vi "SVFA Get Tone Amplitude and Phase (1 Ch).vi"(0 "complex spectrum":T8={"complex spectrum response"={"f0"=0.0, "df"=1.0, "complex spectrum"=[]}, "spectrum info"={"channel name"="", "description"="", "x-axis units"=0, "spectral info"={"spectrum type"=enum."Power [Magnitude^2]", "linear/dB"=enum."linear", "window"=0, "window size"=0, "FFT size"=0}, "engineering units"=0, "custom label"="", "dB reference [EU]"=0.0, "peak units"=enum."rms", "weighting filter"=0, "spectral density?"=FALSE, "unit label"="", "spectrum skewed?"=FALSE, "complimentary spectrum units"=enum."none"}} {"spectrum info"."x-axis units" items=["Time (s)"=0, "Frequency-CB (Hz)"=1, "Frequency-CPB (Hz)"=1248, "Frequency-Arbitrary (Hz)"=2357, "Quefrency (s)"=2, "Revolutions (rev)"=3, "Order"=4, "Speed (RPM)"=11, "Speed (rad/s)"=21, "Index"=65535]; "spectrum info"."weighting filter" items=["Linear", "A-weighting", "B-weighting", "C-weighting", "ITU-R 468-4", "Dolby", "CCITT", "C-message", "Wb", "Wc", "Wd", "We", "Wf", "Wh", "Wj", "Wk", "Wm", "AES17 20 kHz lowpass", "AES17 40 kHz lowpass", "AES17 20 kHz highpass", "AES17 40 kHz highpass"]; "spectrum info"."dB reference [EU]" format="%.2f"; "spectrum info"."engineering units" items=["custom..."=0, "V"=1, "A"=21, "C"=30, "pC"=31, "s"=32, "-"=29, "Pa"=2, "N"=20, "g"=3, "m/s^2"=4, "m/s"=5, "m"=6, "mm/s"=12, "mm"=13, "micron/s"=14, "micron"=15, "in/s^2"=7, "in/s"=8, "in"=9, "mil/s"=10, "mil"=11, "rad/s^2"=16, "rad/s"=17, "rad"=18, "deg/s^2"=26, "deg/s"=27, "deg"=28, "RPM"=22, "cycle/s^2"=23, "Hz"=24, "cycle"=25, "strain"=19]; "spectrum info"."spectral info"."window" items=["None "=0, "Hanning"=1, "Hamming"=2, "Blackman-Harris"=3, "Exact Blackman"=4, "Blackman"=5, "Flat Top"=6, "4 Term B-Harris "=7, "7 Term B-Harris"=8, "Low Sidelobe"=9, "Force - Exponential"=10, "Gaussian"=62]; "complex spectrum response"."complex spectrum" format="%.2f"; "complex spectrum response"."df" format="%.2f"; "complex spectrum response"."f0" format="%.2f"}, 2 "tone frequency [Hz]":dbl=1000.0 format="%.2f", 5 "error in (no error)":errorcluster) -> (14 "identified tone":T1={"frequency [Hz]"=nan, "amplitude [EU pk]"=nan, "phase [deg]"=nan} {"phase [deg]" format="%.2p"; "amplitude [EU pk]" format="%.2p"; "frequency [Hz]" format="%.2f"}, 19 "error out":errorcluster)   [LabVIEW 2017]
doc: "Extracts the value of the spectrum at the specified frequency. Use the frequency coercion control to specify how the frequency should be coerced if it does not exactly coincide with a frequency line. This VI operates on any real-valued spectrum. Wire data to the <B>spectrum</B> input to determine the polymorphic instance to use or manually select the instance."
uses:
  <vilib>/addons/_NISVFA/_Shared subVIs/Controls/svc_Spectrum Info.ctl
  <vilib>/addons/_NISVFA/_Shared subVIs/Controls/svc_X-Axis Units.ctl
  <vilib>/addons/_NISVFA/_Shared subVIs/Controls/svc_Spectrum Type.ctl
  <vilib>/addons/_NISVFA/_Shared subVIs/Controls/svc_Engineering Units Text Ring.ctl
  <vilib>/addons/_NISVFA/_Shared subVIs/Controls/svc_Weighting Filter Text Ring.ctl
  <vilib>/addons/_NISVFA/_Shared subVIs/Controls/svc_Complimentary Spectrum Units.ctl
  <vilib>/addons/_NISVFA/_Spectrum Processing/subVIs/svfa_Window Frequency Response (double array).vi
  <vilib>/Analysis/baseanly.llb/Complex Dot Product.vi
  <vilib>/addons/_NISVFA/_Spectrum Processing/subVIs/svfa_Rect Window Frequency Response.vi
  <vilib>/addons/_NISVFA/_Spectrum Processing/subVIs/svfa_Cosine Window Coefficients.vi
  <vilib>/Analysis/NI_AALBase.lvlib
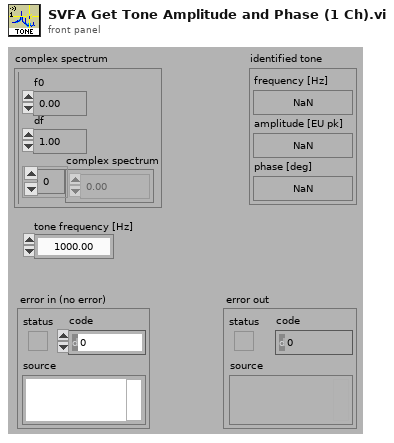
[diagram p1: front panel]
types:
  T1 = cluster{"frequency [Hz]":dbl, "amplitude [EU pk]":dbl, "phase [deg]":dbl}
  T2 = typedef "svc_Spectrum Info.ctl" = cluster{"channel name":string, "description":string, "x-axis units":T3, "spectral info":cluster{"spectrum type":T4, "linear/dB":enum16{"linear", "dB"}, "window":u16, "window size":i32, "FFT size":i32}, "engineering units":T5, "custom label":string, "dB reference [EU]":dbl, "peak units":enum16{"rms", "peak", "peak-peak"}, "weighting filter":T6, "spectral density?":bool, "unit label":string, "spectrum skewed?":bool, "complimentary spectrum units":T7}
  T3 = typedef "svc_X-Axis Units.ctl" = u16
  T4 = typedef "svc_Spectrum Type.ctl" = enum16{"FFT Spectrum [complex]", "Amplitude [Magnitude]", "Power [Magnitude^2]", "Cross Spectrum [complex]", "Frequency Response [Complex]"}
  T5 = typedef "svc_Engineering Units Text Ring.ctl" = u16
  T6 = typedef "svc_Weighting Filter Text Ring.ctl" = u16
  T7 = typedef "svc_Complimentary Spectrum Units.ctl" = enum16{"none", "radians", "degrees", "cycles", "imaginary"}
  T8 = cluster{"complex spectrum response":cluster{"f0":dbl, "df":dbl, "complex spectrum":cdb[]}, "spectrum info":T2}
  T9 = cluster{"frequency [Hz]":dbl, "amplitude":dbl, "phase":dbl}
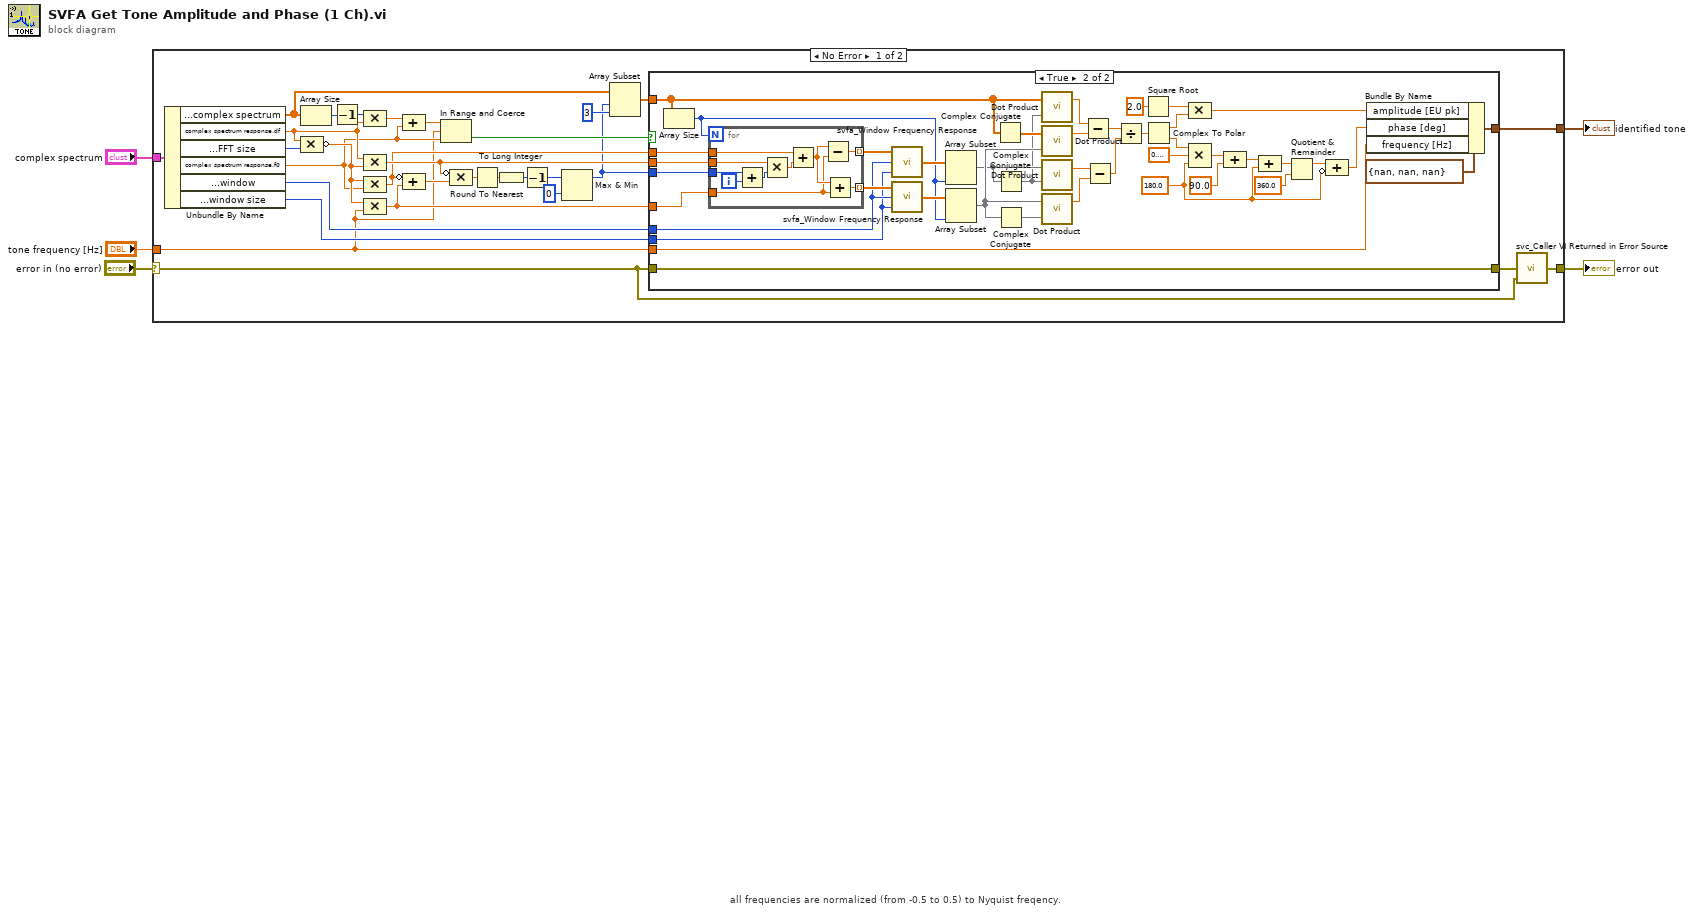
[diagram p0: block diagram]
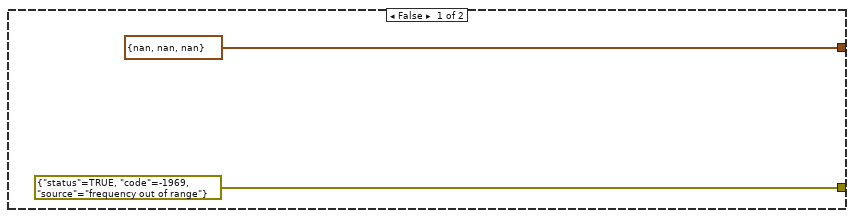
[diagram p2: hidden frame]
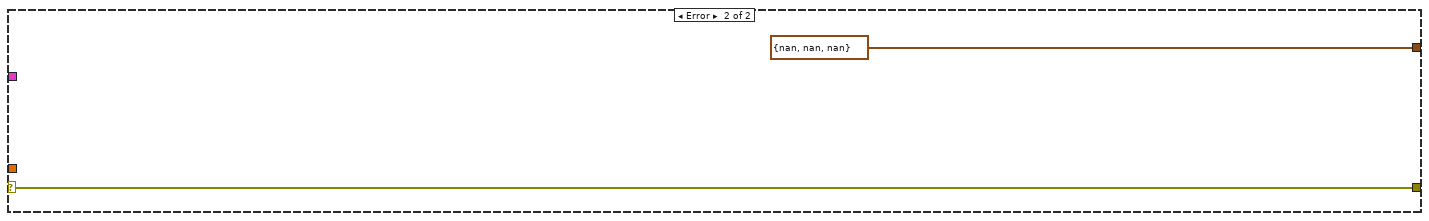
[diagram p3: hidden frame]
diagram:
  # "all frequencies are normalized (from -0.5 to 0.5) to Nyquist freqency."
  n1 = case shown="No Error" "error in (no error)" {
    selector: "error in (no error)" -> [w28 w91]
    tunnel: [w30 w91] -> w5
    tunnel: "complex spectrum" -> [w6 _]
    tunnel: "tone frequency [Hz]" -> [w13 _]
    tunnel: [w27 T9 {"frequency [Hz]"=nan, "amplitude"=nan, "phase"=nan} ("identified tone")] -> w2
    frame No Error {
      n2 = Unbundle By Name(w6) -> ("complex spectrum response.complex spectrum"=w12:cdb[], "complex spectrum response.df"=w18:dbl, "spectrum info.spectral info.FFT size"=w21:i32, "complex spectrum response.f0"=w17:dbl, "spectrum info.spectral info.window"=w15:u16, "spectrum info.spectral info.window size"=w14:i32)
      n3 = Array Size(array=w12) -> (size(s)=w35:i32)
      n4 = Compound Arithmetic op=MULTIPLY(w18, w21) -> (invert w26:dbl)
      n5 = Decrement(x=w35) -> (x-1=w34:i32)
      n6 = Compound Arithmetic op=MULTIPLY(w34, w18) -> (w32:dbl)
      n7 = Compound Arithmetic op=MULTIPLY(w18, w26) -> (w20:dbl)
      n8 = Compound Arithmetic op=MULTIPLY(w26, w17) -> (w19:dbl)
      n9 = Compound Arithmetic op=MULTIPLY(w26, w13) -> (w16:dbl)
      n10 = Compound Arithmetic op=ADD(w32, w17) -> (w31:dbl)
      n11 = Compound Arithmetic op=ADD(invert w19, w16) -> (w22:dbl)
      n12 = In Range and Coerce(upper limit=w31, x=w13, lower limit=w17) -> (In Range?=w33:bool)  [unwired: 1 out]
      n13 = Compound Arithmetic op=MULTIPLY(invert w20, w22) -> (w23:dbl)
      n14 = Round To Nearest(number=w23) -> (nearest integer value=w24:dbl)
      n15 = To Long Integer(number=w24) -> (32bit integer=w25:i32)
      n16 = Decrement(x=w25) -> (x-1=w10:i32)
      n17 = Max & Min(x=w10, y=0) -> (max(x,y)=w7:i32)  [unwired: 1 out]
      n18 = Array Subset(array=w12, index=w7, length=3) -> (w8:cdb[])
      n19 = case shown="True" w33 {
        tunnel: w28 -> [_ w40]
        tunnel: [errorcluster {"status"=TRUE, "code"=-1969, "source"="frequency out of range"} ("error out") w40] -> w29
        tunnel: w13 -> [_ w41]
        tunnel: [T1 {"frequency [Hz]"=nan, "amplitude [EU pk]"=nan, "phase [deg]"=nan} ("identified tone") w57] -> w27
        tunnel: w7 -> [_ w56]
        tunnel: w19 -> [_ w55]
        tunnel: w20 -> [_ w54]
        tunnel: w16 -> [_ w53]
        tunnel: w15 -> [_ w52]
        tunnel: w14 -> [_ w51]
        tunnel: w8 -> [_ w39]
        frame False {
        }
        frame True {
          w43 = 180.0 ("Input")
          n20 = Array Size(array=w39) -> (size(s)=w38:i32)
          n21 = for {
            N: w38 -> [_]
            tunnel: w55 -> [w89]
            tunnel: w54 -> [w83]
            tunnel: w53 -> [w86]
            tunnel: [w85] -> w64 mode=indexing
            tunnel: [w84] -> w65 mode=indexing
            tunnel: w56 -> [w82]
            i -> [w80]
            n22 = Add(x=w82, y=w80) -> (x+y=w81:i32)
            n23 = Multiply(x=w83, y=w81) -> (x*y=w88:dbl)
            n24 = Add(x=w89, y=w88) -> (x+y=w87:dbl)
            n25 = Subtract(x=w87, y=w86) -> (x-y=w85:dbl)
            n26 = Add(x=w87, y=w86) -> (x+y=w84:dbl)
          }
          n27 = call-poly <vilib>:"svfa_Window Frequency Response.vi"("N (window length)"=w51, "window"=w52, "f(normalized)"=w64) -> ("H(f)"=w67:cdb[])
          n28 = call-poly <vilib>:"svfa_Window Frequency Response.vi"("N (window length)"=w51, "window"=w52, "f(normalized)"=w65) -> ("H(f)"=w66:cdb[])
          n29 = Array Subset(array=w67, length=w38) -> (w73:cdb[])  [unwired: 1 in]
          n30 = Array Subset(array=w66, length=w38) -> (w78:cdb[])  [unwired: 1 in]
          n31 = Complex Conjugate(1:w39) -> (0:w72:cdb[])
          n32 = Complex Conjugate(1:w73) -> (0:w71:cdb[])
          n33 = Complex Conjugate(1:w78) -> (0:w70:cdb[])
          n34 = call-poly <vilib>:"Dot Product.vi"("Y Vector"=w71, "X Vector"=w39) -> ("X * Y"=w74:cdb)  [unwired: 1 out]
          n35 = call-poly <vilib>:"Dot Product.vi"("Y Vector"=w78, "X Vector"=w72) -> ("X * Y"=w79:cdb)  [unwired: 1 out]
          n36 = call-poly <vilib>:"Dot Product.vi"("Y Vector"=w71, "X Vector"=w73) -> ("X * Y"=w75:cdb)  [unwired: 1 out]
          n37 = call-poly <vilib>:"Dot Product.vi"("Y Vector"=w70, "X Vector"=w78) -> ("X * Y"=w69:cdb)  [unwired: 1 out]
          n38 = Subtract(x=w74, y=w79) -> (x-y=w76:cdb)
          n39 = Subtract(x=w75, y=w69) -> (x-y=w77:cdb)
          n40 = Divide(x=w76, y=w77) -> (x/y=w68:cdb)
          n41 = Square Root(x=2.0 ("Input")) -> (sqrt(x)=w60:dbl)
          n42 = Complex To Polar(r * e^(i*theta)=w68) -> (r=w62:dbl, theta=w63:dbl)
          n43 = Compound Arithmetic op=MULTIPLY(w60, w62) -> (w58:dbl)
          n44 = Compound Arithmetic op=MULTIPLY(w63, 0.3183098861837907, w43) -> (w49:dbl)
          n45 = Compound Arithmetic op=ADD(w49, 90.0 ("value")) -> (w48:dbl)
          n46 = Compound Arithmetic op=ADD(w48, w43) -> (w47:dbl)
          n47 = Quotient & Remainder(x=w47, y=360.0 ("value")) -> (x-y*floor(x/y)=w45:dbl)  [unwired: 1 out]
          n48 = Compound Arithmetic op=ADD(w45, invert w43) -> (w44:dbl)
          n49 = Bundle By Name(cluster=T1 {"frequency [Hz]"=nan, "amplitude [EU pk]"=nan, "phase [deg]"=nan} ("identified tone"), "amplitude [EU pk]"=w58, "phase [deg]"=w44, "frequency [Hz]"=w41) -> (w57:T1)
        }
      }
      n50 = call <vilib>:"svc_Caller VI Returned in Error Source.vi"("warning input to caller"=w28, "error in (no error)"=w29) -> ("error out"=w30:errorcluster)  [unwired: 3 in]
    }
    frame Error {
    }
  }
  "error out" <- w5
  "identified tone" <- w2
